vi "Parse Query String.vi"(11 "query string":string) -> (3 "Map":map{string, string}(c390))   [LabVIEW 2019, in "Useful HTTP VIs.lvlib"]
uses:
  Useful HTTP VIs/Useful HTTP VIs.lvlib
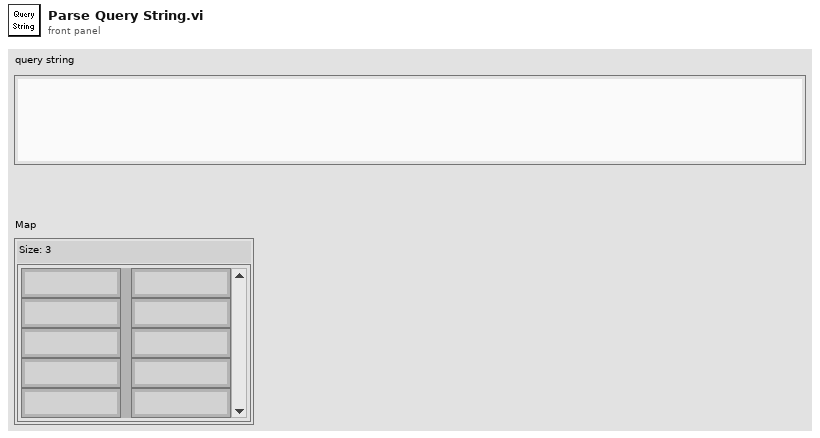
[diagram p1: front panel]
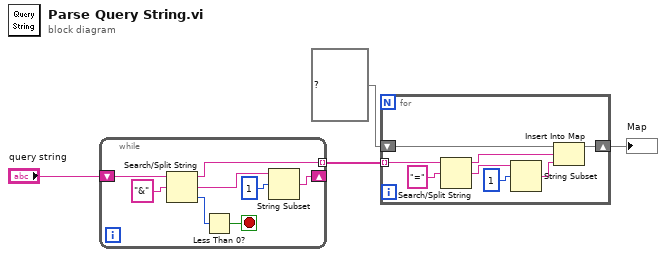
[diagram p0: block diagram]
diagram:
  n1 = while {
    shift-right: [w7] -> _
    shift-left: "query string" -> [w12]
    tunnel: [w10] -> w3 mode=indexing
    stop <- w6 stop-if-true
    n2 = Search/Split String(string=w12, search string/char (-)="&") -> (substring before match=w10:string, match + rest of string=w9:string, offset of match=w5:i32)  [unwired: 1 in]
    n3 = Less Than 0?(x=w5) -> (x < 0?=w6:bool)
    n4 = String Subset(string=w9, offset (0)=1) -> (substring=w7:string)  [unwired: 1 in]
  }
  n5 = for {
    tunnel: w3 -> [w19] mode=indexing
    shift-right: [w13] -> w1
    shift-left: map{string, string} {} ("map") -> [w16]
    n6 = Search/Split String(string=w19, search string/char (-)="=") -> (substring before match=w15:string, match + rest of string=w18:string)  [unwired: 1 in, 1 out]
    n7 = String Subset(string=w18, offset (0)=1) -> (substring=w14:string)  [unwired: 1 in]
    n8 = Insert Into Map(map in=w16, key=w15, value=w14) -> (map out=w13:map{string, string})  [unwired: 2 out]
  }
  "Map" <- w1
